vi "Actor Core.vi"(8 "error in":errorcluster, 11 "Videoscan in":refnum<class "Videoscan.lvclass">) -> (0 "error out":errorcluster, 3 "Actor out":refnum<class "Actor.lvclass">)   [LabVIEW 2014, in "Videoscan.lvclass"]
doc: "(<B>Filename</B>: Actor Framework.lvlib:Actor.lvclass:Actor Core.vi)\n\nReceives messages to the actor, reacts to them, and initiates any error handling that may shut the actor down.\n\nDescendant classes may override this VI to append parallel tasks for the actor to complete while it handles messages. Overrides use the Call Parent Method node."
uses:
  Videoscan.lvclass
  Framework/Hardware/ReadoutDevice/ReadoutDevice.lvclass
  Framework/Interfaces/Viewable Actor/Viewable Actor.lvclass
  Framework/Interfaces/Pipelined Actor/Pipelined Actor Messages/Do Main Action Msg/Do Main Action Msg.lvclass
  <vilib>/ActorFramework/Actor/Actor.lvclass
  Framework/Model/Data/Data2D/Data2D.lvclass
  Framework/Interfaces/Observable Actor/Observable Actor.lvclass
panel:
  out "Stop":bool=TRUE
  out "Preview":dbl[][](graph)
  out "isShow":bool=TRUE
  in  "Read":bool
  in  "Frequency":dbl=100.0
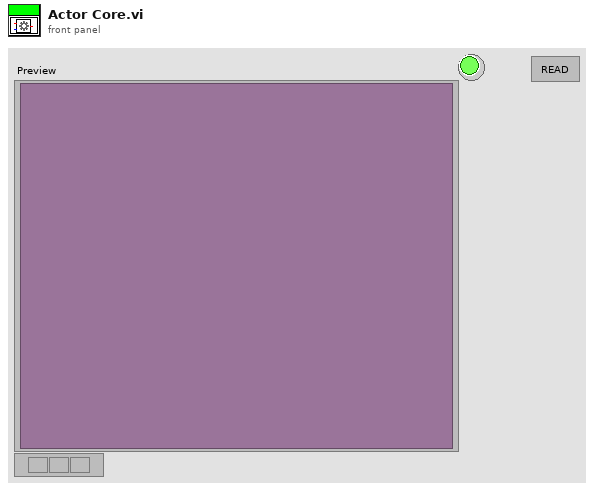
[diagram p1: front panel]
types:
  T1 = typedef "Observable Actor.lvlib/Observable Actor.lvclass/Observer.ctl" = refnum<queue>
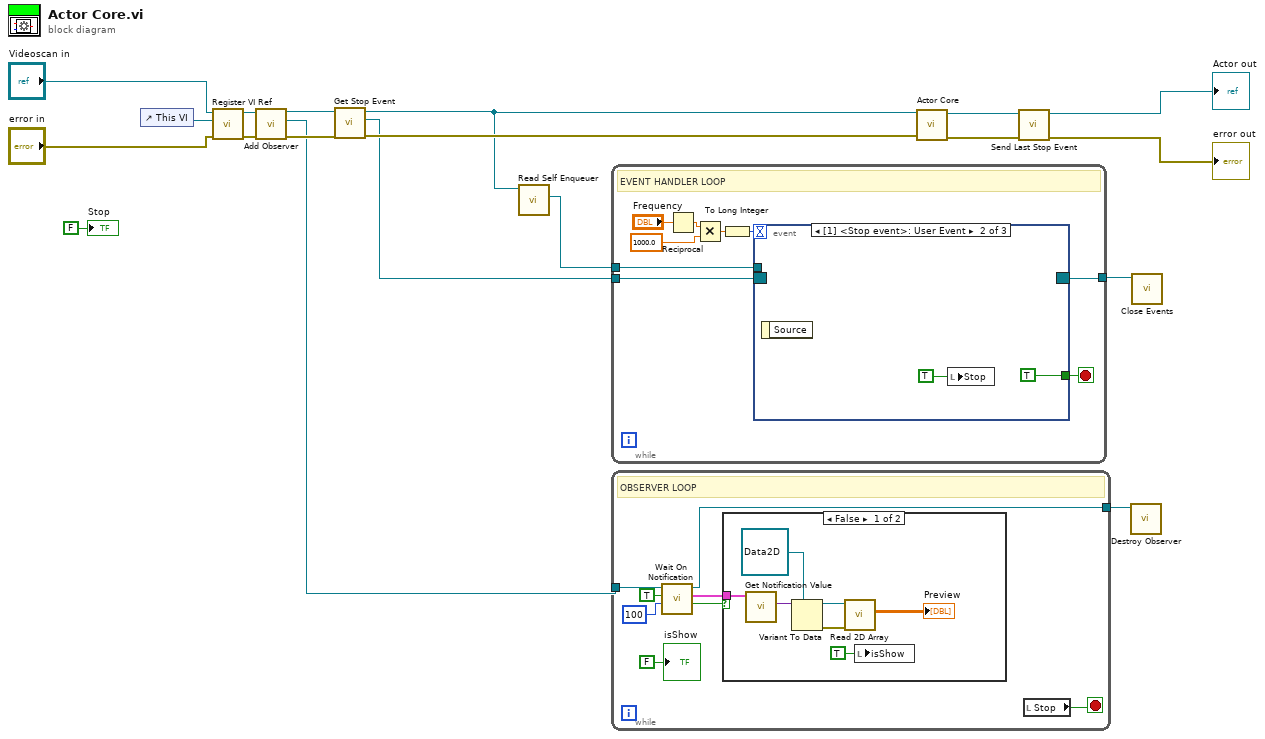
[diagram p0: block diagram]
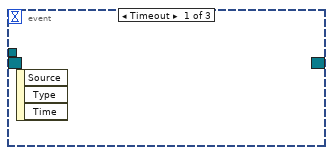
[diagram p3: hidden frame]
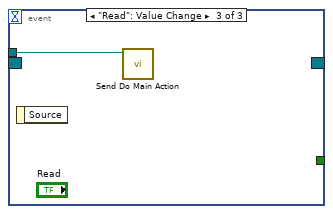
[diagram p4: hidden frame]
diagram:
  n1 = control-ref of="This VI"() -> (w18:refnum<vi>)
  n2 = call "Register VI Ref.vi"("error in (no error)"="error in", "VI ref"=w18, "Viewable Actor in"="Videoscan in") -> ("error out"=w15:errorcluster, "Viewable Actor out"=w16:refnum<class "Videoscan.lvclass">)  [unwired: 7 in]
  n3 = call-dynamic "Add Observer.vi"("error in (no error)"=w15, "Observable Actor in"=w16) -> ("error out"=w19:errorcluster, "new observer"=w14:T1, "Observable Actor out"=w13:refnum<class "Videoscan.lvclass">)  [unwired: 7 in]
  n4 = call-dynamic "Get Stop Event.vi"("error in (no error)"=w19, "Observable Actor in"=w13) -> ("error out"=w12:errorcluster, "Events"=w11:refnum<event-registration>, "Observable Actor out"=w5:refnum<class "Videoscan.lvclass">)  [unwired: 7 in]
  n5 = call <vilib>:"Read Self Enqueuer.vi"("Actor"=w5) -> ("Self Enqueuer"=w17:refnum<class "Message Enqueuer.lvclass">)  [unwired: 10 in]
  n6 = while {
    tunnel: w11 -> [w28]
    tunnel: w17 -> [w27]
    tunnel: [w26] -> w10
    stop <- w25 stop-if-true
    # "EVENT HANDLER LOOP"
    n7 = Reciprocal(x="Frequency") -> (1/x=w23:dbl)
    n8 = Multiply(x=w23, y=1000.0) -> (x*y=w21:dbl)
    n9 = To Long Integer(number=w21) -> (32bit integer=w20:i32)
    n10 = event shown="[1] <Stop event>: User Event" {
      selector: w28 -> [_ _ _]
      dyn-events: [_ _ _] -> w26
      timeout: w20 -> [_ _ _]
      tunnel: w27 -> [_ _ w31]
      tunnel: [_ TRUE _] -> w25
      event Timeout {
        n11 = event-data() -> ()  [unwired: 1 in, 3 out]
      }
      event User Event {
        n12 = event-data() -> ()  [unwired: 1 in, 1 out]
        n13 = local write "Stop"(TRUE ("Stop")) -> ()
      }
      event "Read": Value Change {
        n14 = event-data() -> ()  [unwired: 1 in, 1 out]
        n15 = call "Send Do Main Action.vi"("Message Enqueuer"=w31) -> ()  [unwired: 9 in, 2 out]
      }
    }
  }
  n16 = while {
    tunnel: w14 -> [w34]
    tunnel: [w33] -> w7
    stop <- w39 stop-if-true
    # "OBSERVER LOOP"
    n17 = call "Wait On Notification.vi"("timeout in ms (-1)"=100, "ignore previous (F)"=TRUE, "observer in"=w34) -> ("timed out?"=w35:bool, "notification"=w36:cluster{"value":variant, "name":string}, "observer out"=w33:T1)  [unwired: 5 in, 1 out]
    n18 = case shown="False" w35 {
      tunnel: w36 -> [w46 _]
      frame False {
        n19 = call "Get Notification Value.vi"("notification in"=w46) -> ("data"=w45:variant)  [unwired: 7 in, 1 out]
        n20 = Variant To Data(type=refnum<class "Data2D.lvclass"> refnum ("Data2D.lvclass"), Variant=w45) -> (data=w42:refnum<class "Data2D.lvclass">, error out=w41:errorcluster)  [unwired: 1 in]
        n21 = call "Read 2D Array.vi"("error in (no error)"=w41, "Data2D in"=w42) -> ("2D Array"=→"Preview":dbl[][])  [unwired: 7 in, 2 out]
        n22 = local write "isShow"(TRUE ("isShow")) -> ()
      }
      frame True {
      }
    }
    n23 = local read "Stop"() -> (w39:bool)
    "isShow" <- FALSE ("Boolean")
  }
  n24 = call-parent "Actor Core.vi"("error in"=w12, "Actor in"=w5) -> ("error out"=w8:errorcluster, "Actor out"=w9:refnum<class "Actor.lvclass">)  [unwired: 8 in]
  n25 = call "Send Last Stop Event.vi"("error in (no error)"=w8, "Actor in"=w9) -> ("error out"=→"error out":errorcluster, "Actor  out"=→"Actor out":refnum<class "Actor.lvclass">)  [unwired: 8 in]
  n26 = call "Destroy Observer.vi"("observer in"=w7) -> ()  [unwired: 11 in]
  n27 = call "Close Events.vi"("events"=w10) -> ()  [unwired: 11 in]
  "Stop" <- FALSE ("Stop")
